vi "WaitOnSync.vi"(8 "error in (no error)":errorcluster, 9 "Enable":bool=TRUE, 11 "ControlState in":T1 {"ChainMask" format="0x%02x"}) -> (0 "error out":errorcluster, 3 "ControlState out":T1 {"ChainMask" format="0x%02x"})   [LabVIEW 2020, in "ArduinoSerialBling.lvlib"]
uses:
  Documents/Robotics/swerve-template/Swerve Robot Project Template/LEDs/Implementation/ArduinoSerialBling.lvlib
  ControlState.ctl
  ChainState.ctl
  <vilib>/Instr/_visa.llb/VISA Flush IO Buffer Mask.ctl
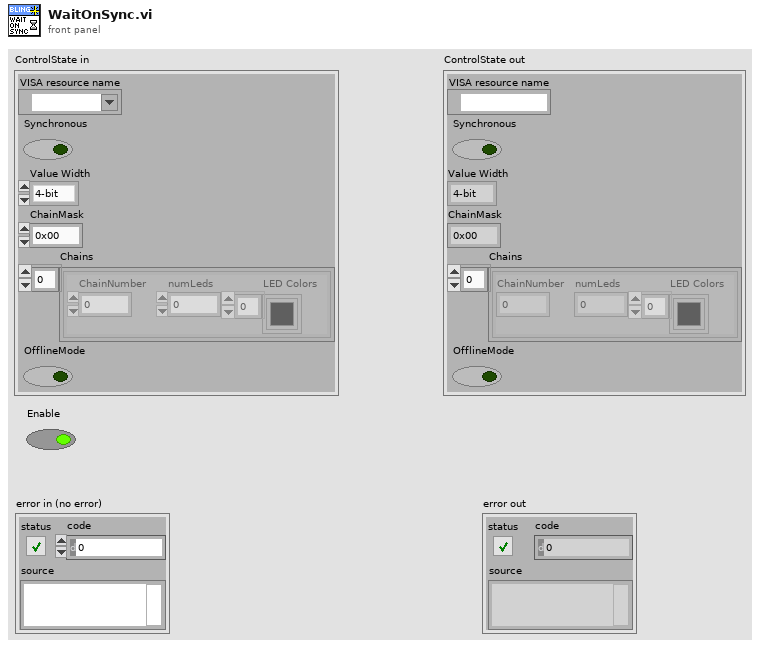
[diagram p1: front panel]
types:
  T1 = typedef "ArduinoSerialBling.lvlib/ControlState.ctl" = cluster{"VISA resource name":refnum<visa-resource-name>, "Synchronous":bool, "Value Width":enum16{"4-bit", "8-bit"}, "ChainMask":u8, "Chains":T2[], "OfflineMode":bool}
  T2 = typedef "ArduinoSerialBling.lvlib/ChainState.ctl" = cluster{"ChainNumber":u8, "numLeds":u8, "LED Colors":u32[]}
  T3 = typedef "VISA Flush IO Buffer Mask.ctl" = u16
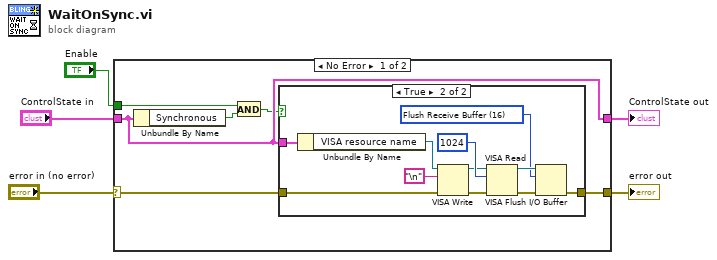
[diagram p0: block diagram]
diagram:
  n1 = case shown="No Error" "error in (no error)" {
    selector: "error in (no error)" -> [w11 w25]
    tunnel: [w10 w25] -> w4
    tunnel: "ControlState in" -> [w9 w24]
    tunnel: [w9 w24] -> w2
    tunnel: "Enable" -> [w7 _]
    frame No Error {
      n2 = Unbundle By Name(w9) -> ("Synchronous"=w6:bool)
      n3 = And(x=w7, y=w6) -> (x .and. y?=w8:bool)
      n4 = case shown="True" w8 {
        tunnel: w11 -> [w12 w14]
        tunnel: [w12 w20] -> w10
        tunnel: w9 -> [_ w18]
        frame False {
        }
        frame True {
          w21 = T3 16 items=["Flush Receive Buffer"=16, "Write Transmit Buffer to Device"=32, "Flush Receive Buffer (No I/O)"=64, "Flush Transmit Buffer"=128] ("Mask")
          n5 = Unbundle By Name(w18) -> ("VISA resource name"=w17:refnum<visa-resource-name>)
          n6 = VISA Write(VISA resource name=w17, write buffer="\n", error in (no error)=w14) -> (VISA resource name out=w13:refnum<visa-resource-name>, error out=w15:errorcluster)  [unwired: 1 out]
          n7 = VISA Read(VISA resource name=w13, byte count=u32 1024, error in (no error)=w15) -> (VISA resource name out=w23:refnum<visa-resource-name>, error out=w22:errorcluster)  [unwired: 2 out]
          n8 = VISA Flush I/O Buffer(VISA resource name=w23, mask (16)=w21, error in (no error)=w22) -> (error out=w20:errorcluster)  [unwired: 1 out]
        }
      }
    }
    frame Error {
    }
  }
  "ControlState out" <- w2
  "error out" <- w4
